vi "WS1050 AD7747 READ.vi"(8 "error in":errorcluster, 9 "Log (T)":bool, 11 "DUT Mask Mode (All)":T1=enum."All") -> (0 "error out":errorcluster, 3 "AD7747 Values":string[][](table))   [LabVIEW 2012]
uses:
  Type Defs/WSVCAP SHL I2C DUT Mask Mode Enum.ctl
panel:
  # "Single Read 900A22"
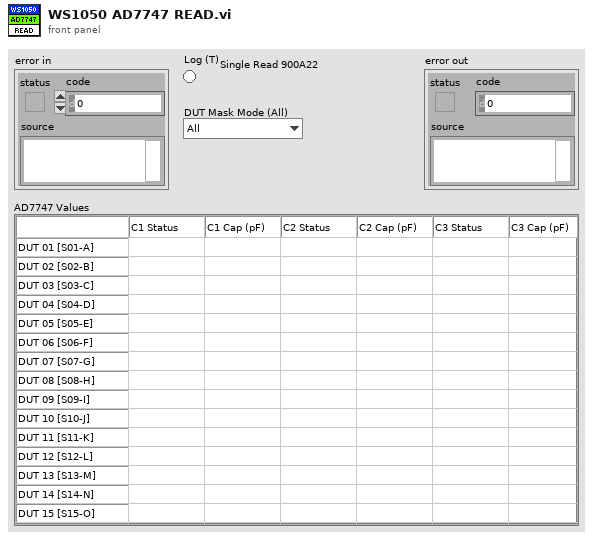
[diagram p1: front panel]
types:
  T1 = typedef "WSVCAP SHL I2C DUT Mask Mode Enum.ctl" = enum16{"Custom", "C1", "C2", "C3", "All"}
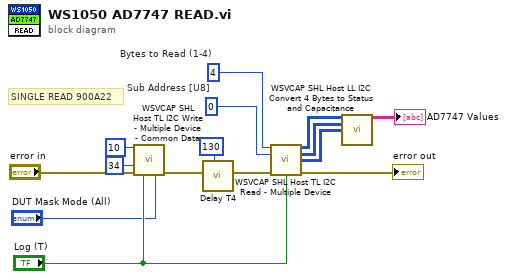
[diagram p0: block diagram]
diagram:
  w13 = u8 4  # Bytes to Read (1-4)
  w14 = u8 0  # Sub Address [U8]
  # "SINGLE READ 900A22"
  n1 = call "WSVCAP SHL Host TL I2C Write - Multiple Device - Common Data.vi"("Sub Address"=u8 10, "Data Out [U8]"=u8 34, "error in"="error in", "Log (T)"="Log (T)", "DUT Mask Mode (All)"="DUT Mask Mode (All)") -> ("error out"=w4:errorcluster)  [unwired: 10 in]
  n2 = call "Delay T4.vi"("milliseconds to wait"=u32 130, "error in (no error)"=w4) -> ("error out"=w5:errorcluster)  [unwired: 9 in]
  n3 = call "WSVCAP SHL Host TL I2C Read - Multiple Device.vi"("Bytes to Read (1-4)"=w13, "Sub Address [U8]"=w14, "error in"=w5, "Log (T)"="Log (T)") -> ("C1:1-16 Read Data [U8]"=w12:u8[][], "C2:1-16 Read Data [U8]"=w11:u8[][], "C3:1-16 Read Data [U8]"=w9:u8[][], "error out"=→"error out":errorcluster)  [unwired: 8 in]
  n4 = call "WSVCAP SHL Host LL I2C Convert 4 Bytes to Status and Capacitance.vi"("C1:1-16 Read Data [U8]"=w12, "C2_1-16 Read Data [U8]"=w11, "C3_1-16 Read Data [U8]"=w9) -> ("AD7747 Values"=→"AD7747 Values":string[][])  [unwired: 12 in]
